vi "pp2_log_DAQconfig.vi"(10 "refnum in":refnum<file>, 11 "Daq config":T1={"Sound AO"="Dev2/ao0", "Shock intesity AO"="Dev2/ao1", "Code_LED DO"="Dev2/port1:2", "Switch DI"="Dev2/port0/line0:1", "Webcam"="cam9", "Sound AO task"="", "Sound card task"=0, "Shock intensity AO task"="", "Code_LED DO task"="", "Switch DI task"="", "AO <=> Sound card"=FALSE, "Sound card"=0, "sample rate"=8000.0, "Variable shock"=FALSE, "Webcam on"=TRUE, "Tone gate PFI"="/Dev2/PFI1", "Waveform memo"={"t0"=timestamp(0 s since 1904-01-01), "dt"=1.0, "Y"=[]}} {"sample rate" min=8000.0; "Sound card task" format="%.0x"}) -> (2 "refnum out":refnum<file>)   [LabVIEW 2013]
uses:
  pp2_CTL_DaqConfig.ctl
  <vilib>/userdefined/High Color/IMAQdx.ctl
  <vilib>/sound2/lvsound2.llb/Sound Output Task ID.ctl
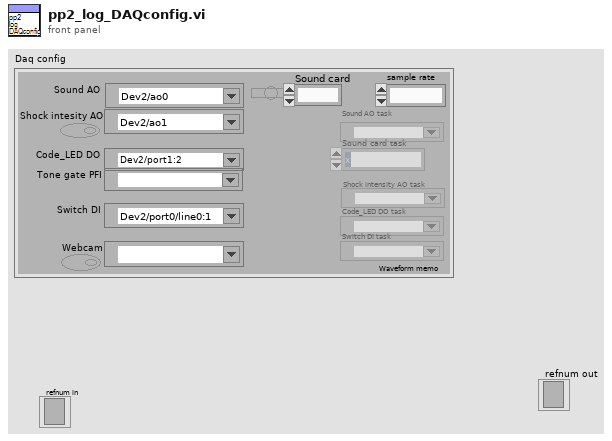
[diagram p1: front panel]
types:
  T1 = typedef "pp2_CTL_DaqConfig.ctl" = cluster{"Sound AO":tag, "Shock intesity AO":tag, "Code_LED DO":tag, "Switch DI":tag, "Webcam":T2, "Sound AO task":refnum<k21>, "Sound card task":T3, "Shock intensity AO task":refnum<k21>, "Code_LED DO task":refnum<k21>, "Switch DI task":refnum<k21>, "AO <=> Sound card":bool, "Sound card":u32, "sample rate":dbl, "Variable shock":bool, "Webcam on":bool, "Tone gate PFI":tag, "Waveform memo":waveform(dbl)}
  T2 = typedef "IMAQdx.ctl" = refnum<k21>
  T3 = typedef "Sound Output Task ID.ctl" = u32
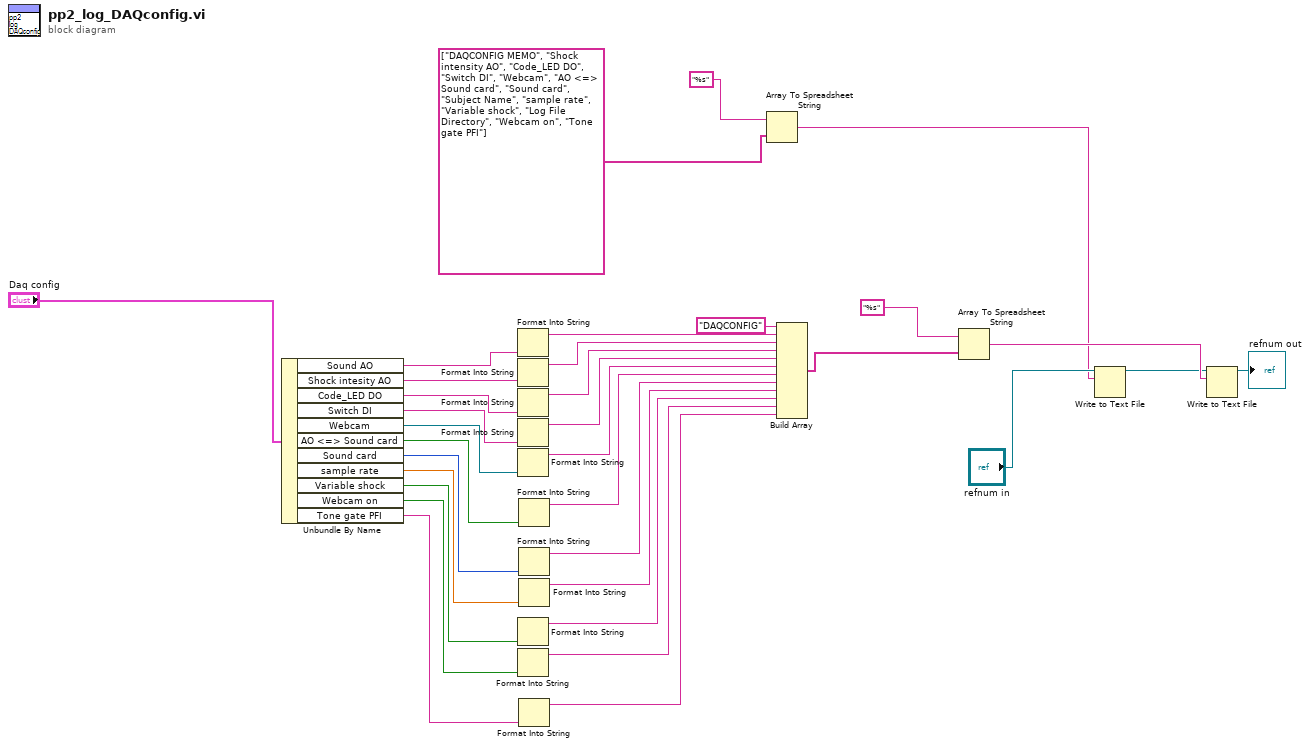
[diagram p0: block diagram]
diagram:
  n1 = Unbundle By Name("Daq config") -> ("Sound AO"=w33:tag, "Shock intesity AO"=w29:tag, "Code_LED DO"=w28:tag, "Switch DI"=w27:tag, "Webcam"=w26:T2, "AO <=> Sound card"=w25:bool, "Sound card"=w19:u32, "sample rate"=w18:dbl, "Variable shock"=w17:bool, "Webcam on"=w16:bool, "Tone gate PFI"=w15:tag)
  n2 = Format Into String(w33) -> (resulting string=w31:string)  [unwired: 3 in, 1 out]
  n3 = Format Into String(w29) -> (resulting string=w24:string)  [unwired: 3 in, 1 out]
  n4 = Format Into String(w28) -> (resulting string=w23:string)  [unwired: 3 in, 1 out]
  n5 = Format Into String(w27) -> (resulting string=w22:string)  [unwired: 3 in, 1 out]
  n6 = Format Into String(w26) -> (resulting string=w21:string)  [unwired: 3 in, 1 out]
  n7 = Format Into String(w17) -> (resulting string=w12:string)  [unwired: 3 in, 1 out]
  n8 = Format Into String(w16) -> (resulting string=w11:string)  [unwired: 3 in, 1 out]
  n9 = Format Into String(w25) -> (resulting string=w20:string)  [unwired: 3 in, 1 out]
  n10 = Format Into String(w19) -> (resulting string=w14:string)  [unwired: 3 in, 1 out]
  n11 = Format Into String(w18) -> (resulting string=w13:string)  [unwired: 3 in, 1 out]
  n12 = Format Into String(w15) -> (resulting string=w10:string)  [unwired: 3 in, 1 out]
  n13 = Array To Spreadsheet String(array=string[] ["DAQCONFIG MEMO", "Shock intensity AO", "Code_LED DO", "Switch DI", "Webcam", "AO <=> Sound card", "Sound card", "Subject Name", "sample rate", "Variable shock", "Log File Directory", "Webcam on", "Tone gate PFI"], 3:"%s" ("format string")) -> (spreadsheet string=w1:string)  [unwired: 1 in]
  n14 = Build Array("DAQCONFIG" ("element"), w31, w24, w23, w22, w21, w20, w14, w13, w12, w11, w10) -> (w7:string[])
  n15 = Array To Spreadsheet String(array=w7, 3:"%s" ("format string")) -> (spreadsheet string=w8:string)  [unwired: 1 in]
  n16 = Write to Text File(file (use dialog)="refnum in", text=w1) -> (refnum out=w3:refnum<file>)  [unwired: 2 in, 2 out]
  n17 = Write to Text File(file (use dialog)=w3, text=w8) -> (refnum out=→"refnum out":refnum<file>)  [unwired: 2 in, 2 out]
